vi "FGV Gasteilerkorrektur.vi"(0 "Abweichung":sgl[][](array[numeric]) format="%#_5g", 5 "Bevesnummer":string[](array[string]), 7 "Aktiv":bool, 9 "Gültigkeit bis":timestamp[](array[timestamp]) format="%<%Y/%m/%d>T", 11 "Gasteiler":enum16{"1", "2"}(ring), 12 "Aktion":T1) -> (3 "Vereinzelt":sgl[](array[numeric]), 4 "Abweichung":sgl[][](array[numeric]), 6 "Bevesnummer":string[](array[string]), 8 "Aktiv":bool, 10 "Gültigkeit bis":timestamp[](array[timestamp]), 15 "Gasteiler":enum16{"1", "2"}(ring))   [LabVIEW 2020, in "Linearisierung v2.lvlib" / "Gasteiler.lvlib"]
uses:
  Gasteiler.lvlib
  Aktion FGV Gasteiler Korrektur.ctl
  Allgemein/allgemeine Sub-VIs.lvlib
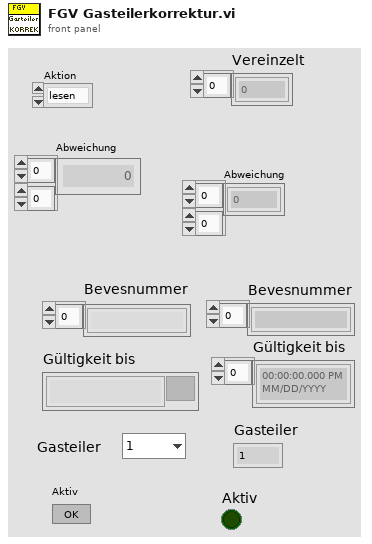
[diagram p1: front panel]
types:
  T1 = typedef "Linearisierung v2.lvlib/Gasteiler.lvlib/Aktion FGV Gasteiler Korrektur.ctl" = enum16{"lesen", "schreiben", "laden", "speichern", "B-nr und Gültig", "Gasteilernr.", "Vereinzeln", "aktiv"}
  T2 = cluster{"Abweichung":sgl[][], "Bevesnummer":string[], "Gültigkeit bis":timestamp[], "Gasteiler":enum16{"1", "2"}, "Aktiv":bool}
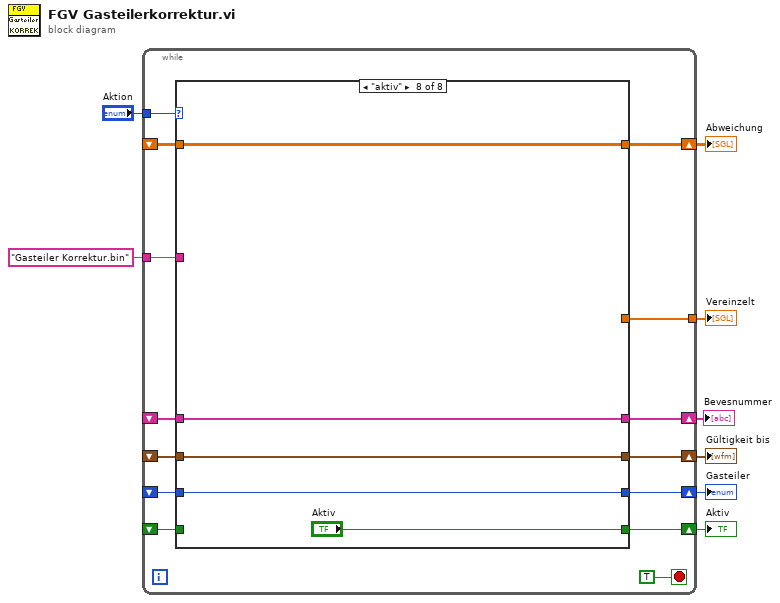
[diagram p0: block diagram]
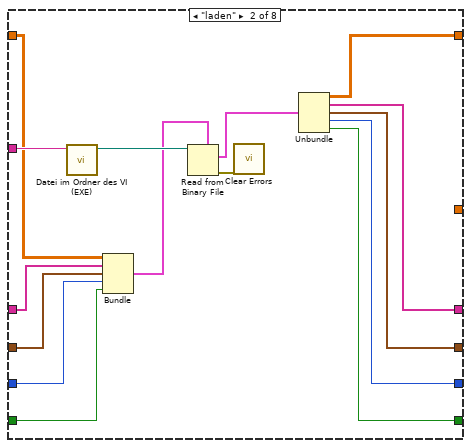
[diagram p3: hidden frame]
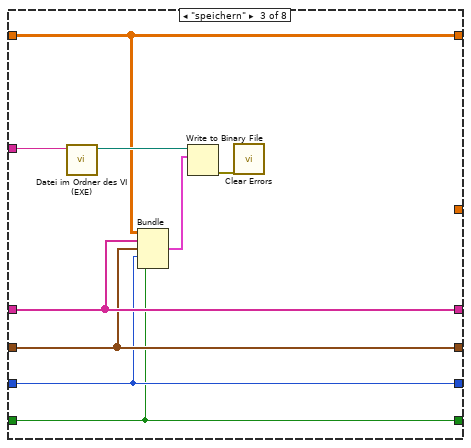
[diagram p4: hidden frame]
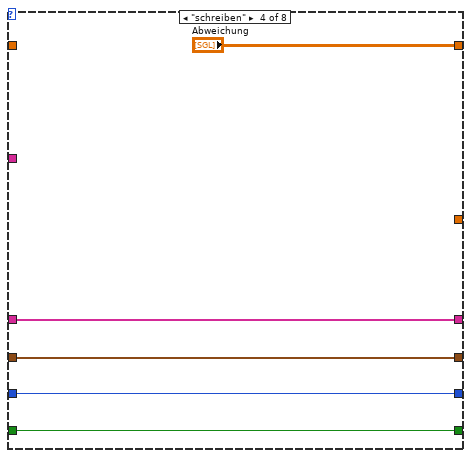
[diagram p5: hidden frame]
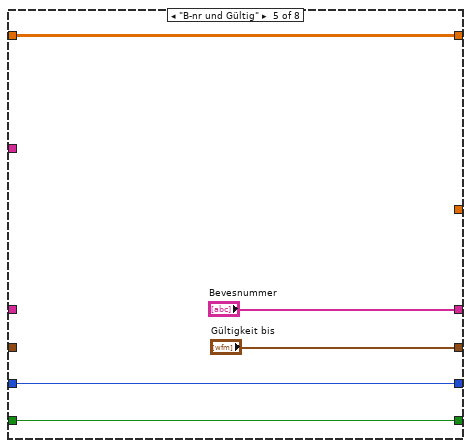
[diagram p6: hidden frame]
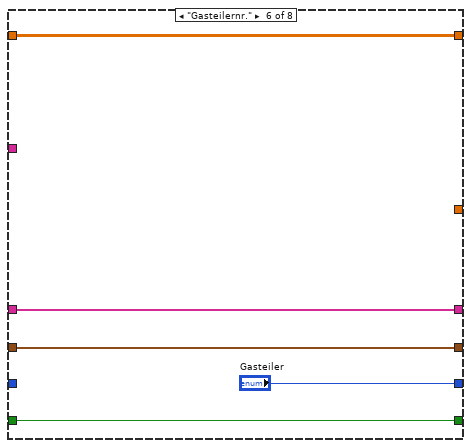
[diagram p7: hidden frame]
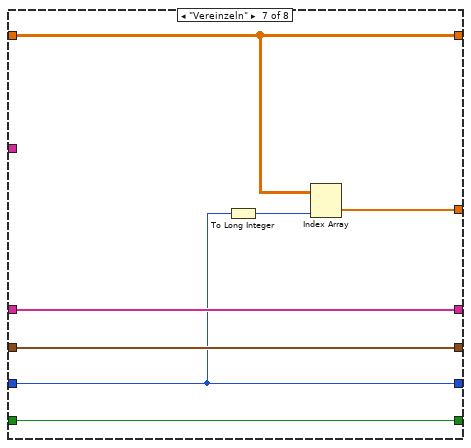
[diagram p8: hidden frame]
diagram:
  n1 = while {
    tunnel: "Aktion" -> [w21]
    shift-right: [w20] -> w7
    shift-left: _ -> [w19]
    tunnel: "Gasteiler Korrektur.bin" ("Dateiname") -> [w18]
    shift-right: [w16] -> w3
    shift-left: _ -> [w14]
    shift-right: [w17] -> w5
    shift-left: _ -> [w15]
    shift-right: [w13] -> w4
    shift-left: _ -> [w12]
    tunnel: [w11] -> w2
    shift-right: [w10] -> w1
    shift-left: _ -> [w9]
    stop <- TRUE stop-if-true
    n2 = case shown="\"aktiv\"" w21 {
      tunnel: [w27 w33 w48 "Abweichung" w60 w66 w71 w78] -> w20
      tunnel: w19 -> [w27 w39 w48 _ w60 w66 w71 w78]
      tunnel: w18 -> [_ w42 w51 _ _ _ _ _]
      tunnel: [w26 w32 w47 w55 "Bevesnummer" w64 w73 w77] -> w17
      tunnel: [w25 w31 w46 w54 "Gültigkeit bis" w63 w72 w76] -> w16
      tunnel: w15 -> [w26 w38 w47 w55 _ w64 w73 w77]
      tunnel: w14 -> [w25 w37 w46 w54 _ w63 w72 w76]
      tunnel: [w24 w30 w45 w53 w59 "Gasteiler" w70 w75] -> w13
      tunnel: w12 -> [w24 w36 w45 w53 w59 _ w70 w75]
      tunnel: [_ _ _ _ _ _ w69 _] -> w11
      tunnel: [w23 w28 w43 w52 w57 w62 w67 "Aktiv"] -> w10
      tunnel: w9 -> [w23 w29 w43 w52 w57 w62 w67 _]
      frame "lesen", Default {
      }
      frame "laden" {
        n3 = call "Datei im Ordner des VI (EXE).vi"("Dateiname"=w42) -> ("Dateipfad im Ordner des Haupt-VIs"=w41:path)  [unwired: 8 in, 2 out]
        n4 = Bundle("Abweichung"=w39, "Bevesnummer"=w38, "Gültigkeit bis"=w37, "Gasteiler"=w36, "Aktiv"=w29) -> (w35:T2)  [unwired: 1 in]
        n5 = Read from Binary File(5:w35, 11:w41) -> (0:w40:errorcluster, 2:w34:T2)  [unwired: 4 in, 2 out]
        n6 = call <vilib>:"Clear Errors.vi"("error in (no error)"=w40) -> ()  [unwired: 5 in, 2 out]
        n7 = Unbundle(w34) -> ("Abweichung"=w33:sgl[][], "Bevesnummer"=w32:string[], "Gültigkeit bis"=w31:timestamp[], "Gasteiler"=w30:enum16{"1", "2"}, "Aktiv"=w28:bool)
      }
      frame "speichern" {
        n8 = call "Datei im Ordner des VI (EXE).vi"("Dateiname"=w51) -> ("Dateipfad im Ordner des Haupt-VIs"=w50:path)  [unwired: 8 in, 2 out]
        n9 = Bundle("Abweichung"=w48, "Bevesnummer"=w47, "Gültigkeit bis"=w46, "Gasteiler"=w45, "Aktiv"=w43) -> (w44:T2)  [unwired: 1 in]
        n10 = Write to Binary File(file (use dialog)=w50, data=w44) -> (error out=w49:errorcluster)  [unwired: 4 in, 2 out]
        n11 = call <vilib>:"Clear Errors.vi"("error in (no error)"=w49) -> ()  [unwired: 5 in, 2 out]
      }
      frame "schreiben" {
      }
      frame "B-nr und Gültig" {
      }
      frame "Gasteilernr." {
      }
      frame "Vereinzeln" {
        n12 = To Long Integer(number=w70) -> (32bit integer=w68:i32)
        n13 = Index Array(array=w71, index (col)=w68) -> (element=w69:sgl[])  [unwired: 1 in]
      }
      frame "aktiv" {
      }
    }
  }
  "Abweichung" <- w7
  "Bevesnummer" <- w5
  "Gasteiler" <- w4
  "Gültigkeit bis" <- w3
  "Vereinzelt" <- w2
  "Aktiv" <- w1
